vi "Dashboard Main.vi"() -> ()   [LabVIEW 2014]
uses:
  <vilib>/event_ctls.llb/eventvkey.ctl
  <vilib>/Rock Robotics/Network Tables/SD Write Number.vi
  <vilib>/Rock Robotics/WPI/Dashboard/WPI_DashboardLogging Global.vi
  <vilib>/Rock Robotics/Network Tables/SD Read Number.vi
  <vilib>/Utility/config.llb/Write Key (String).vi
  <vilib>/Utility/config.llb/Write Key (I32).vi
  <vilib>/Utility/config.llb/NI_LVConfig.lvlib
panel:
  in  "TCP":refnum<k5>
  in  "Rec Mode":enum32{"Stop", "Record", "Playback"}(radio)
  in  "Vision":u16(ring) items=["Camera Off", "USB Camera SW", "USB Camera HW", "IP Camera"]
  out "Camera IP":string
  out "Image Message":string="Timeout in Camera Communications"
  in  "Dashboard Tab":T1(tab)
  in  "Camera Settings":T2={"Frame Rate"=30, "Compression"=30, "Size"=1} {"Frame Rate" scale=1.0..30.0; "Size" items=["640x480", "320x240", "160x120"]}
  out "MotorChart R":cluster{"Numeric":dbl, "Numeric":dbl}(graph)
  out "MotorChart L":T3(graph)
  out "MotorSliders R":cluster{"MotorSlide1":dbl, "MotorSlide2":dbl} {"MotorSlide2" scale=-1.0..1.0 scale format="%#_2e"; "MotorSlide1" scale=-1.0..1.0 scale format="%#_2e"}
  out "MotorSliders L":T4 {"MotorSlide4 2" scale=0.0..14.0 scale format="%#_2e"; "MotorSlide2" scale=-1.0..1.0 scale format="%#_2e"; "MotorSlide1" scale=-1.0..1.0 scale format="%#_2e"}
  out "Gyro":dbl(knob) scale=0.0..360.0
  out "JS1 Z":dbl(slide) scale=-1.0..1.0 scale format="%#_2e"
  out "JS1 Graph":cluster{"X":dbl, "Y":dbl}[](graph)
  out "JS1 Buttons":T5
  out "JS2 Z":dbl(slide) scale=-1.0..1.0 scale format="%#_2e"
  out "JS2 Graph":cluster{"X":dbl, "Y":dbl}[](graph)
  out "JS2 Buttons":T5
  out "Mode":T6(ring)=enum."Auto Disabled"
  in  "DB Camera Config":bool
  out "fps":dbl format="%#.1g"
  out "Mbps":dbl format="%#.1g"
  out "Mbps 2":bool
  in  "DB/String 9":string
  in  "DB/String 8":string
  in  "DB/String 7":string
  in  "DB/String 6":string
  in  "DB/String 5":string
  in  "DB/String 4":string
  in  "DB/String 3":string
  in  "DB/String 2":string
  in  "DB/String 1":string
  in  "DB/String 0":string
  in  "DB/Slider 0":dbl(slide) scale=0.0..5.0
  in  "DB/Slider 1":dbl(slide) scale=0.0..5.0
  in  "DB/Slider 2":dbl(slide) scale=0.0..5.0
  in  "DB/Slider 3":dbl(slide) scale=0.0..5.0
  out "DB/LED 3":bool
  out "DB/LED 2":bool
  out "DB/LED 1":bool
  out "DB/LED 0":bool
  in  "DB/Button 3":bool
  in  "DB/Button 2":bool
  in  "DB/Button 1":bool
  in  "DB/Button 0":bool caption="New Name"
  out "Guide Box":bool
  in  "a/b":bool
  out "Lift up?":bool
  out "Clasper open?":bool
  out "Clasper closed?":bool
  out "Lift down?":bool
  in  "Autonomous":i32(listbox)
  out "Encoder":dbl(slide) scale=-1.0..1.0 scale format="%#_2e"
  out "Cam Pan":dbl(slide) scale=-1.0..1.0 scale format="%#_2e"
  out "Lift":dbl(slide) scale=-1.0..1.0 scale format="%#_2e"
  out "Cam Tilt":dbl(slide) scale=-1.0..1.0 scale format="%#_2e"
  out "Clasper":dbl(slide) scale=-1.0..1.0 scale format="%#_2e"
  in  "Test Slider":dbl(slide) scale=0.0..100.0 scale format="%#_3g"
  in  "On/Off":bool caption="Solenoid"
  in  "Test Name":u16(ring) items=["Select the test to run...", "Example Test", "-------------------------------", "List of tests is built in robot code.", "Replace with your own automated tests."]
  in  "Test Tree":string(tree)
  in  "Motor":cluster{"Value":dbl, "Enable":bool} {"Value" scale=-1.0..1.0 scale format="%#_3g"}
  out "Progress":T7 {"Test Progress" scale=0.0..100.0}
  in  "Rev/Fwd":cluster{"Forward":bool, "Reverse":bool}
  in  "Test Ring":u16(ring) items=["Monochrome", "Color"]
  in  "Listbox":i32(listbox)
  out "Tree":string(tree)
  out "Camera Image":T8(plugin-control)
  out "Boolean":bool
  # "Left"
  # "Front"
  # "Right"
  # "Battery"
  # "Encoder"
  # "Cam Pan"
  # "Lift"
  # "Cam Tilt"
  # "Clasper"
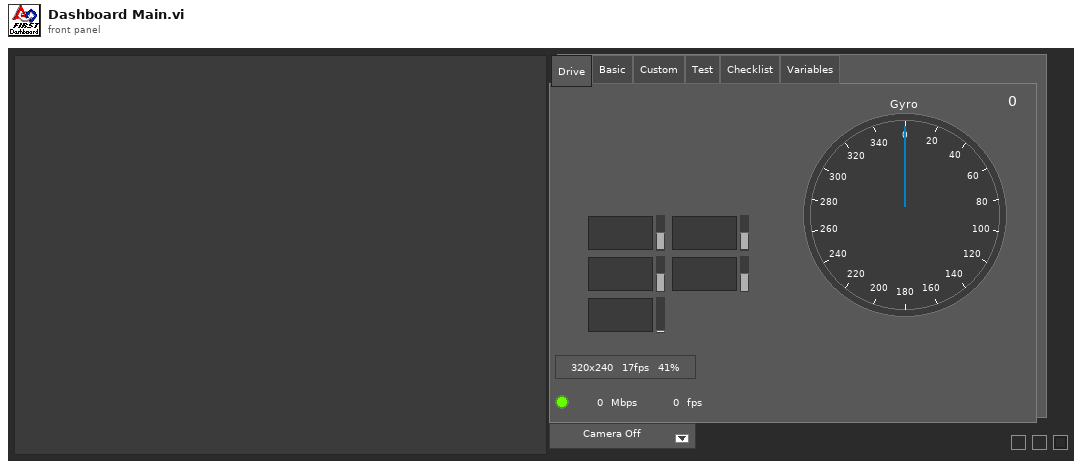
[diagram p1: front panel]
types:
  T1 = enum32{"Drive", "Basic", "Custom", "Test", "Checklist", "Variables"}
  T2 = cluster{"Frame Rate":i32, "Compression":i32, "Size":u16}
  T3 = cluster{"Numeric":dbl, "Numeric":dbl, "Battery V":dbl}
  T4 = cluster{"MotorSlide1":dbl, "MotorSlide2":dbl, "MotorSlide4 2":dbl}
  T5 = cluster{bool, bool, bool, bool, bool, bool, bool, bool, bool, bool, bool, bool}
  T6 = enum8{"Tele-Op Disabled", "Tele-Op Enabled", "Auto Disabled", "Auto Enabled", "Test Disabled", "Test Enabled", "Disconnected", "No Code", "E-Stop"}
  T7 = cluster{"Test Progress":u8, "Test Progress Text":string}
  T8 = typedef "IMAQ Image.ctl" = refnum<image>
  T9 = typedef "Image Type" = u32
  T10 = cluster{"Camera Image":refnum<vi>, "Dashboard Tab":refnum<vi>, "Boolean":refnum<vi>, "Vision":refnum<vi>, "Rec Mode":refnum<vi>, "Test Slider":refnum<vi>, "On/Off ":refnum<vi>, "Test Ring":refnum<vi>, "Rev/Fwd":refnum<vi>, "Test Name":refnum<vi>, "Motor":refnum<vi>, "Progress":refnum<vi>, "CheckList":refnum<vi>, "Tree":refnum<vi>, "Test Tree":refnum<vi>}
  T11 = cluster{"Error Strings":string, "Disable Counts":cluster{u16, u16}, "Rail Faults":cluster{u16, u16, u16}, "Robot IP":string, "DB Mode":u8, "Event Info":cluster{"Name":string, "Type":u8, "Number":u16, "Replay":u8}, "Camera Addr":string}
  T12 = cluster{"Storage":cluster{"Disk Free":u64, "RAM Block":u32, "RAM free":u32}, "CPU Utilization":cluster{"CPU % ISR":sgl, "CPU % Time Crit":sgl, "CPU % Timed Str":sgl, "CPU % High":sgl, "CPU % Above":sgl, "CPU % Normal":sgl, "CPU % Low":sgl}, "CAN":cluster{"% Bus Utilization":sgl, "Bus Off Cnt":u32, "TX_FIFO Full Cnt":u32, "Receive Error Cnt":u8, "Transmit Error Cnt":u8}, "HID":cluster{"HID Outputs":u32, "Rumble Low":u16, "Rumble High":u16}[]}
  T13 = cluster{"Status bits":cluster{"Test Mode":bool, "Autonomous":bool, "Enabled":bool, "Code Start":bool, "Brownout":bool, "Reserved 2":bool, "Reserved 3":bool, "E-Stop":bool}, "Code Trace":cluster{"Disabled":bool, "TeleOp":bool, "Auto":bool, "Test":bool}, "Controller Type":enum16{"unknown", "cRIO", "roboRio"}, "Code?":enum16{"unknown", "noCode", "code"}, "Battery V":dbl}
  T14 = cluster{"Control Bits":cluster{"TestMode":bool, "Autonomous":bool, "Enabled":bool, "FMS Present":bool, bool, bool, bool, "E-Stop":bool}, "Team Station ":u8, "Countdown":sgl, "Joystick Values":cluster{"Axes":dbl[], "Buttons":bool[], "POVs":i16[]}[]}
  T15 = cluster{"Axes":dbl[], "Buttons":bool[], "POVs":i16[]}[]
  T16 = cluster{"Axes":dbl[], "Buttons":bool[], "POVs":i16[]}
  T17 = cluster{"Buttons[0]":bool, "Buttons[1]":bool, "Buttons[2]":bool, "Buttons[3]":bool, "Buttons[4]":bool, "Buttons[5]":bool, "Buttons[6]":bool, "Buttons[7]":bool, "Buttons[8]":bool, "Buttons[9]":bool, "Buttons[10]":bool, "Buttons[11]":bool}
  T18 = typedef "NI_LVConfig.lvlib/Config Data RefNum.ctl" = refnum<k1>
  T19 = cluster{"Operation":enum16{"Update", "Clear"}, "Color Box":u32}[]
  T20 = typedef "eventvkey.ctl" = enum16{"ASCII", "Enter", "Return", "Shift", "Ctrl", "Alt", "Cmd", "Opt", "Caps", "NumLock", "Clear", "Break", "Up", "Down", "Left", "Right", "Insert", "Delete", "Home", "End", "PageUp", "PageDown", "Escape", "Help", "Pause", "ScrollLock", "F1", "F2", "F3", "F4", "F5", "F6", "F7", "F8", "F9", "F10", "F11", "F12", "F13", "F14", "F15", "F16", "F17", "F18", "F19", "F20", "F21", "F22", "F23", "F24", "Play", "VolumeUp", "VolumeDown", "Mute", "Two Byte Char"}
  T21 = cluster{"Image Size":bool, "Image Type":bool, "Pixel Value":bool, "ROI Information":bool, "Zoom Factor":bool}
  T22 = enum8{"Enabled", "Disabled", "Disabled and Grayed Out"}
  T23 = cluster{"Operation":enum16{"Update", "Clear"}, "Color Box":u32}
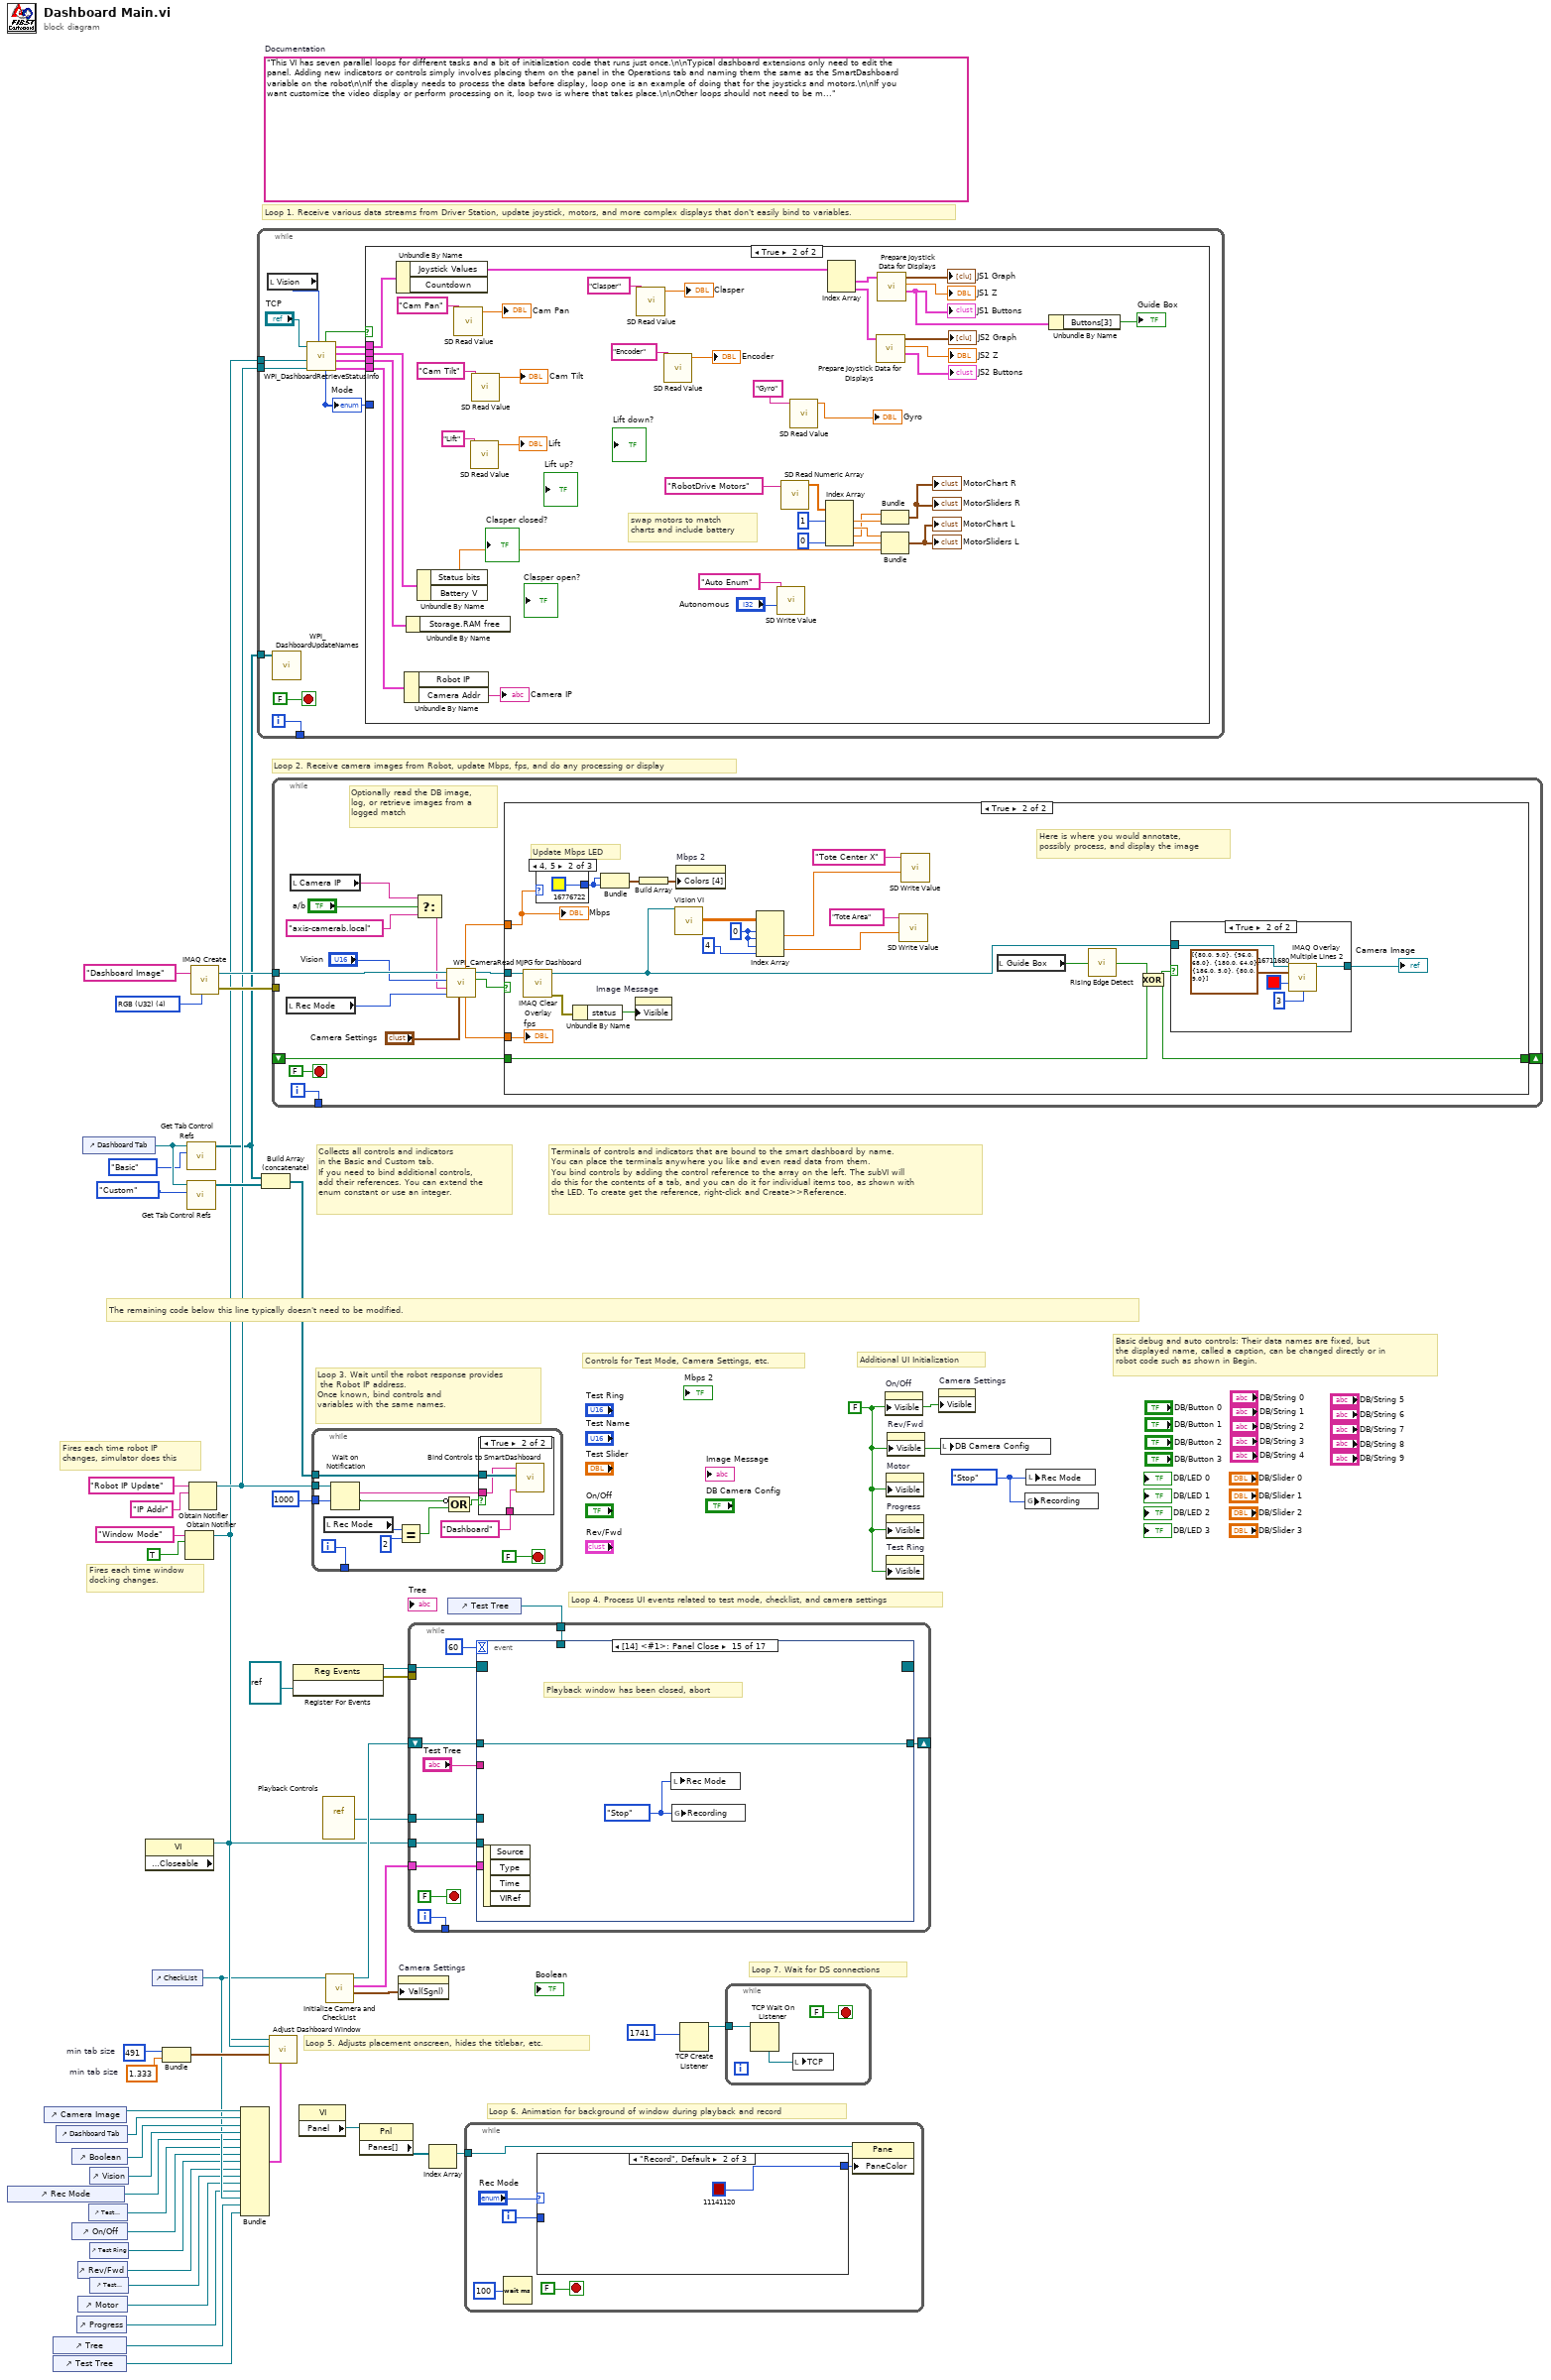
[diagram p0: block diagram]
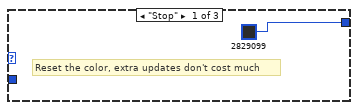
[diagram p3: hidden frame]
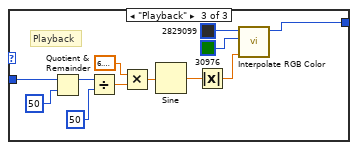
[diagram p4: hidden frame]
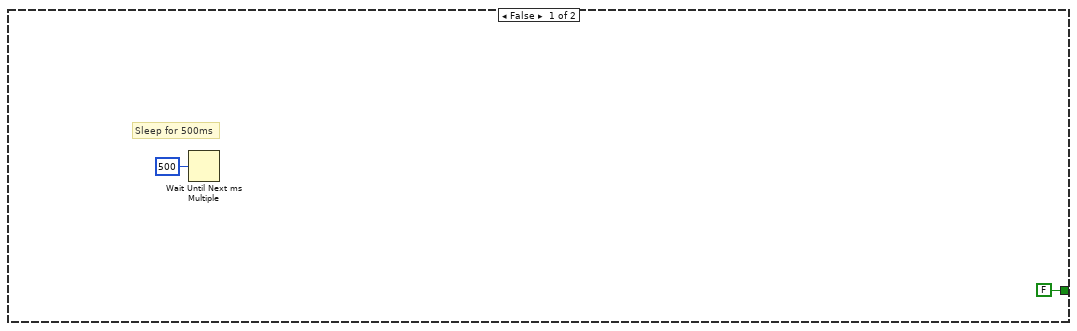
[diagram p6: hidden frame]
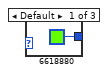
[diagram p8: hidden frame]
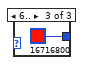
[diagram p9: hidden frame]
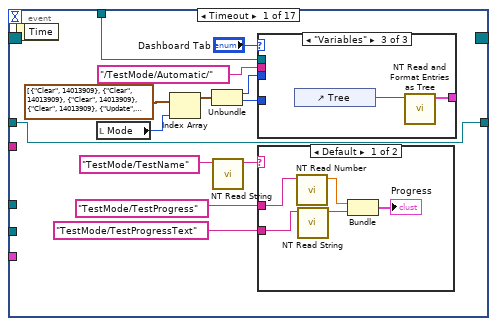
[diagram p10: hidden frame]
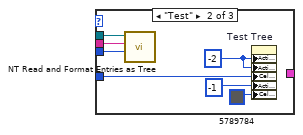
[diagram p12: hidden frame]
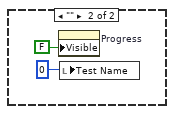
[diagram p13: hidden frame]
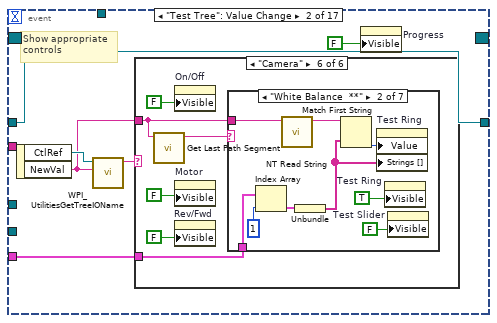
[diagram p14: hidden frame]
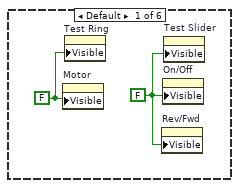
[diagram p15: hidden frame]
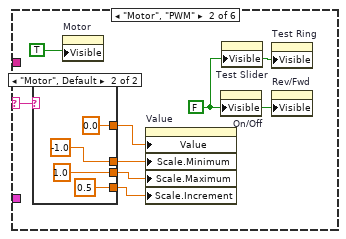
[diagram p16: hidden frame]
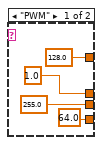
[diagram p17: hidden frame]
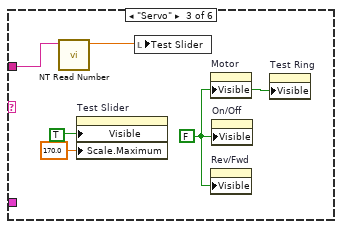
[diagram p18: hidden frame]
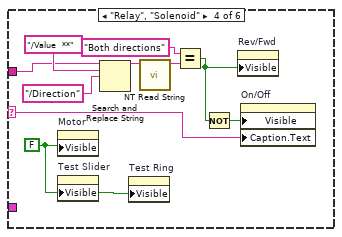
[diagram p19: hidden frame]
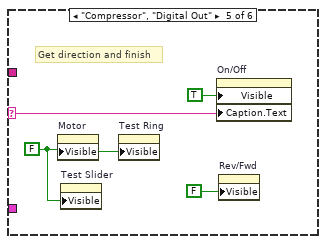
[diagram p20: hidden frame]
diagram:
  w24 = 491  # min tab size
  w23 = 1.333  # min tab size
  w32 = enum32{"Stop", "Record", "Playback"}."Stop" ("Rec Mode")
  w6 = FALSE ("Visible")
  (unwired) "This VI has seven parallel loops for different tasks and a bit of initialization code that runs just once.\n\nTypical dashboard extensions only need to edit the panel. Adding new indicators or controls simply involves placing them on the panel in the Operations tab and naming them the same as the SmartDashboard variable on the robot\n\nIf the display needs to process the data before display, loop one is an example of doing that for the joysticks and motors.\n\nIf you want customize the video display or perform processing on it, loop two is where that takes place.\n\nOther loops should not need to be modified. They are pretty standard, and document the task they perform."  # Documentation
  w52 = T9 4 items=["Grayscale (U8)", "Grayscale (I16)", "Grayscale (SGL)", "Complex (CSG)", "RGB (U32)", "HSL (U32)", "RGB (U64)"] ("Image Type")
  # "Loop 7. Wait for DS connections"
  # "Basic debug and auto controls: Their data names are fixed, but\nthe displayed name, called a caption, can be changed directly or in\nrobot code such as shown in Begin."
  # "Controls for Test Mode, Camera Settings, etc."
  # "Additional UI Initialization"
  # "Loop 6. Animation for background of window during playback and record"
  # "Fires each time robot IP\nchanges, simulator does this"
  # "Fires each time window\ndocking changes."
  # "Collects all controls and indicators\nin the Basic and Custom tab.\nIf you need to bind additional controls,\nadd their references. You can extend the\nenum constant or use an integer."
  # "The remaining code below this line typically doesn't need to be modified."
  # "Loop 4. Process UI events related to test mode, checklist, and camera settings"
  # "Terminals of controls and indicators that are bound to the smart dashboard by name.\nYou can place the terminals anywhere you like and even read data from them.\nYou bind controls by adding the control reference to the array on the left. The subVI will\ndo this for the contents of a tab, and you can do it for individual items too, as shown with\nthe LED. To create get the reference, right-click and Create>>Reference."
  # "Loop 3. Wait until the robot response provides\n the Robot IP address.\nOnce known, bind controls and\nvariables with the same names."
  # "Loop 5. Adjusts placement onscreen, hides the titlebar, etc."
  # "Loop 1. Receive various data streams from Driver Station, update joystick, motors, and more complex displays that don't easily bind to variables."
  # "Loop 2. Receive camera images from Robot, update Mbps, fps, and do any processing or display"
  n1 = control-ref of="Rec Mode"() -> (w12:refnum<vi>)
  n2 = control-ref of="Camera Image"() -> (w27:refnum<vi>)
  n3 = control-ref of="Tree"() -> (w16:refnum<vi>)
  n4 = control-ref of="Test Tree"() -> (w15:refnum<vi>)
  n5 = control-ref of="Dashboard Tab"() -> (w26:refnum<vi>)
  n6 = control-ref of="Boolean"() -> (w21:refnum<vi>)
  n7 = control-ref of="On/Off"() -> (w10:refnum<vi>)
  n8 = control-ref of="Progress"() -> (w7:refnum<vi>)
  n9 = control-ref of="Rev/Fwd"() -> (w8:refnum<vi>)
  n10 = control-ref of="Motor"() -> (w13:refnum<vi>)
  n11 = control-ref of="Dashboard Tab"() -> (w30:refnum<vi>)
  n12 = control-ref of="Test Slider"() -> (w11:refnum<vi>)
  n13 = control-ref of="Vision"() -> (w25:refnum<vi>)
  n14 = control-ref of="Test Ring"() -> (w9:refnum<vi>)
  n15 = control-ref of="Test Name"() -> (w14:refnum<vi>)
  n16 = property class="VI" props=["Front Panel.Closeable"]() -> (reference out=w31:refnum<vi>)  [unwired: 2 in, 2 out]
  n17 = control-ref of="CheckList"() -> (w17:refnum<vi>)
  n18 = Bundle("min tab size"=w24, "min tab size"=w23) -> (w22:cluster{"min tab size":i32, "min tab size":dbl})  [unwired: 1 in]
  n19 = Obtain Notifier(name (unnamed)="Window Mode", notification data type=TRUE) -> (notifier out=w3:refnum<notifier>)  [unwired: 2 in, 2 out]
  n20 = call <vilib>:"Get Tab Control Refs.vi"("Page Index"=T1."Basic" ("Dashboard Tab"), "TabControl in"=w30) -> ("ControlsOnPage"=w4:refnum<vi>[])  [unwired: 9 in]
  n21 = call <vilib>:"Get Tab Control Refs.vi"("Page Index"=T1."Custom" ("Dashboard Tab"), "TabControl in"=w30) -> ("ControlsOnPage"=w29:refnum<vi>[])  [unwired: 9 in]
  n22 = Obtain Notifier(name (unnamed)="Robot IP Update", notification data type="IP Addr" ("name (unnamed)")) -> (notifier out=w5:refnum<notifier>)  [unwired: 2 in, 2 out]
  n23 = call "IMAQ Create"("Image Name"="Dashboard Image", "Image Type"=w52) -> ("New Image"=w50:T8, "error out"=w49:errorcluster)  [unwired: 2 in, 1 out]
  n24 = Bundle("Camera Image"=w27, "Dashboard Tab"=w26, "Boolean"=w21, "Vision"=w25, "Rec Mode"=w12, "Test Slider"=w11, "On/Off"=w10, "Test Ring"=w9, "Rev/Fwd"=w8, "Test Name"=w14, "Motor"=w13, "Progress"=w7, "CheckList"=w17, "Tree"=w16, "Test Tree"=w15) -> (w18:T10)  [unwired: 1 in]
  n25 = while {
    tunnel: [w64] -> _
    tunnel: w5 -> [w58]
    tunnel: w4 -> [w57]
    tunnel: w3 -> [w53]
    i -> [w64]
    stop <- FALSE stop-if-true
    n26 = local read "Vision"() -> (w55:u16)
    n27 = call <vilib>:"WPI_DashboardUpdateNames.vi"("Controls on Tab"=w57) -> ()  [unwired: 11 in]
    n28 = call <vilib>:"WPI_DashboardRetrieveStatusInfo.vi"("Vision"=w55, "Binding Refnum"=w58, "Window Mode Notifier"=w53, "TCP Cnx"="TCP") -> ("Power and Errors"=w59:T11, "Robot Metrics"=w62:T12, "Status Info"=w63:T13, "Control Info"=w60:T14, "Robot Mode"=w56:T6, "Process?"=w61:bool)  [unwired: 2 in]
    "Mode" <- w56
    n29 = case shown="True" w61 {
      tunnel: w63 -> [_ w105]
      tunnel: w62 -> [_ w104]
      tunnel: w60 -> [_ w103]
      tunnel: w59 -> [_ w102]
      tunnel: w56 -> [_ _]
      frame False {
      }
      frame True {
        # "swap motors to match\ncharts and include battery"
        n30 = Unbundle By Name(w103) -> ("Joystick Values"=w81:T15)  [unwired: 1 out]
        n31 = Unbundle By Name(w102) -> ("Camera Addr"=→"Camera IP":string)  [unwired: 1 out]
        n32 = Unbundle By Name(w104) -> ()  [unwired: 1 out]
        n33 = Unbundle By Name(w105) -> ("Battery V"=w92:dbl)  [unwired: 1 out]
        n34 = call-poly <vilib>:"SD Read Value.vi"("Name"="Cam Pan") -> ("Numeric"=→"Cam Pan":dbl)  [unwired: 8 in, 2 out]
        n35 = call-poly <vilib>:"SD Read Value.vi"("Name"="Lift") -> ("Numeric"=→"Lift":dbl)  [unwired: 8 in, 2 out]
        n36 = call-poly <vilib>:"SD Read Value.vi"("Name"="Cam Tilt") -> ("Numeric"=→"Cam Tilt":dbl)  [unwired: 8 in, 2 out]
        n37 = call-poly <vilib>:"SD Read Value.vi"("Name"="Clasper") -> ("Numeric"=→"Clasper":dbl)  [unwired: 8 in, 2 out]
        n38 = call-poly <vilib>:"SD Read Value.vi"("Name"="Encoder") -> ("Numeric"=→"Encoder":dbl)  [unwired: 8 in, 2 out]
        n39 = call-poly <vilib>:"SD Write Value.vi"("Numeric"="Autonomous", "Name"="Auto Enum") -> ()  [unwired: 8 in, 2 out]
        n40 = call <vilib>:"SD Read Numeric Array.vi"("Name"="RobotDrive Motors") -> ("Numeric Array"=w80:dbl[])  [unwired: 8 in, 2 out]
        n41 = call-poly <vilib>:"SD Read Value.vi"("Name"="Gyro") -> ("Numeric"=→"Gyro":dbl)  [unwired: 8 in, 2 out]
        n42 = Index Array(array=w80, index #1=1, index #4=0) -> (element #1=w97:dbl, element #2=w98:dbl, element #3=w96:dbl, element #4=w101:dbl)  [unwired: 2 in]
        n43 = Index Array(array=w81) -> (element #1=w91:T16, element #2=w87:T16)  [unwired: 2 in]
        n44 = call "Prepare Joystick Data for Displays.vi"("Joystick Values"=w87) -> ("Buttons"=→"JS2 Buttons":T17, "Z Axis"=→"JS2 Z":dbl, "Cartesian Data"=→"JS2 Graph":cluster{"X axis":dbl, "X axis":dbl}[])  [unwired: 8 in]
        n45 = call "Prepare Joystick Data for Displays.vi"("Joystick Values"=w91) -> ("Buttons"=w66:T17, "Z Axis"=→"JS1 Z":dbl, "Cartesian Data"=→"JS1 Graph":cluster{"X axis":dbl, "X axis":dbl}[])  [unwired: 8 in]
        "JS1 Buttons" <- w66
        n46 = Bundle("Numeric"=w96, "Numeric"=w97) -> (→"MotorChart R" →"MotorSliders R":cluster{"Numeric":dbl, "Numeric":dbl})  [unwired: 1 in]
        n47 = Bundle("Numeric"=w98, "Numeric"=w101, "Battery V"=w92) -> (→"MotorChart L" →"MotorSliders L":T3)  [unwired: 1 in]
        n48 = Unbundle By Name(w66) -> ("Buttons[3]"=→"Guide Box":bool)
      }
    }
  }
  n49 = Build Array (concatenate)(w4, w29) -> (w28:refnum<vi>[])
  n50 = call "Adjust Dashboard Window.vi"("Sizing Refnums"=w18, "Size Constraints"=w22, "VI"=w31, "Notifier in"=w3) -> ()  [unwired: 8 in]
  n51 = while {
    tunnel: w50 -> [w119]
    tunnel: w49 -> [_]
    tunnel: [w120] -> _
    shift-right: [w107] -> _
    shift-left: _ -> [w106]
    i -> [w120]
    stop <- FALSE stop-if-true
    # "Optionally read the DB image,\nlog, or retrieve images from a\nlogged match"
    n52 = local read "Rec Mode"() -> (w113:enum32{"Stop", "Record", "Playback"})
    n53 = local read "Camera IP"() -> (w109:string)
    n54 = Select(t=w109, s="a/b", f="axis-camerab.local") -> (s? t:f=w108:string)
    n55 = call <vilib>:"WPI_CameraRead MJPG for Dashboard.vi"("Camera Settings"="Camera Settings", "Rec Mode"=w113, "Camera IP"=w108, "Camera Mode"="Vision", "Refnum in"=w119) -> ("Active"=w117:bool, "Refnum out"=w118:T8, "FPS"=w116:dbl, "Bandwidth (Mbps)"=w115:dbl)  [unwired: 3 in]
    n56 = case shown="True" w117 {
      tunnel: w118 -> [_ w139]
      tunnel: w115 -> [_ w138]
      tunnel: w116 -> [_ w137]
      tunnel: [FALSE w129] -> w107
      tunnel: w106 -> [_ w125]
      frame False {
        # "Sleep for 500ms"
        n57 = Wait Until Next ms Multiple(millisecond multiple=u32 500) -> ()  [unwired: 1 out]
      }
      frame True {
        w131 = 0 ("disabled index (row)")
        # "Here is where you would annotate,\npossibly process, and display the image"
        # "Update Mbps LED"
        n58 = call "IMAQ Clear Overlay"("Image"=w139) -> ("error out"=w143:errorcluster, "Image Out"=w124:T8)  [unwired: 2 in, 7 out]
        n59 = case shown="4, 5" w138 {
          tunnel: [u32 6618880 ("Color Box") u32 16776722 ("Color Box") u32 16716800 ("Color Box")] -> w140
          frame Default {
          }
          frame 4, 5 {
          }
          frame 6.. {
          }
        }
        n60 = Unbundle By Name(w143) -> ("status"=w144:bool)
        n61 = Bundle("Color Box"=w140, "Color Box"=w140) -> (w142:cluster{"Color Box":u32, "Color Box":u32})  [unwired: 1 out]
        n62 = property on="Image Message" class="Str"("Visible"=w144) -> ()  [unwired: 2 in, 2 out]
        n63 = Build Array(w142) -> (w141:cluster{"Color Box":u32, "Color Box":u32}[])
        n64 = call "Vision VI.vi"("Image In"=w124) -> ("Particle Measurements (Pixels)"=w136:dbl[][])  [unwired: 24 in, 2 out]
        n65 = property on="Mbps 2" class="Bool (strict)"("Colors [4]"=w141) -> ()  [unwired: 2 in, 2 out]
        n66 = Index Array(array=w136, index (row) #1=w131, index (col) #1=w131, index (row) #2=w131, index (col) #2=4 ("index (row)")) -> (element #1=w130:dbl, element #2=w133:dbl)
        n67 = call-poly <vilib>:"SD Write Value.vi"("Numeric"=w133, "Name"="Tote Area") -> ()  [unwired: 8 in, 2 out]
        n68 = call-poly <vilib>:"SD Write Value.vi"("Numeric"=w130, "Name"="Tote Center X") -> ()  [unwired: 8 in, 2 out]
        n69 = local read "Guide Box"() -> (w127:bool)
        n70 = call "Rising Edge Detect.vi"("Input"=w127) -> ("Output"=w126:bool)
        n71 = Exclusive Or(1:w125, 2:w126) -> (0:w129:bool)
        n72 = case shown="True" w129 {
          tunnel: [w145 w147] -> w128
          tunnel: w124 -> [w145 w146]
          frame False {
          }
          frame True {
            n73 = call "IMAQ Overlay Multiple Lines 2"("Image"=w146, "Line End Points"=cluster{"X":dbl, "Y":dbl}[] [{"X"=80.0, "Y"=9.0}, {"X"=96.0, "Y"=68.0}, {"X"=180.0, "Y"=64.0}, {"X"=186.0, "Y"=5.0}, {"X"=80.0, "Y"=9.0}], "Color"=u32 16711680, "Width"=u32 3) -> ("Image Out"=w147:T8)  [unwired: 10 in, 1 out]
          }
        }
        "Camera Image" <- w128
        "Mbps" <- w138
        "fps" <- w137
      }
    }
  }
  n74 = register-events(refnum<vi> refnum) -> (reference out=w36:refnum<event-registration>, error out=w35:errorcluster)  [unwired: 2 in]
  n75 = property class="VI"() -> ("Panel"=w39:refnum<vi>)  [unwired: 2 in, 2 out]
  n76 = while {
    tunnel: w28 -> [w165]
    tunnel: w5 -> [w163]
    tunnel: [w161] -> _
    tunnel: u32 1000 ("milliseconds to wait") -> [w160]
    i -> [w161]
    stop <- FALSE stop-if-true
    n77 = local read "Rec Mode"() -> (w156:enum32{"Stop", "Record", "Playback"})
    n78 = Wait on Notification(notifier=w163, timeout in ms (-1)=w160) -> (notification=w162:string, timed out?=w158:bool)  [unwired: 2 in, 2 out]
    n79 = Equal?(x=w156, y=u16 2 ("Rec Mode")) -> (x = y?=w157:bool)
    n80 = Compound Arithmetic op=OR(invert w158, w157) -> (w159:bool)
    n81 = case shown="True" w159 {
      tunnel: w165 -> [_ w168]
      tunnel: w162 -> [_ w167]
      tunnel: "Dashboard" -> [_ w166]
      frame False {
      }
      frame True {
        n82 = call <vilib>:"Bind Controls to SmartDashboard.vi"("Client Name"=w166, "Bound Control Refs"=w168, "Server IP Address"=w167) -> ()  [unwired: 9 in]
      }
    }
  }
  n83 = vi-ref "Playback Controls.vi"() -> (w37:refnum<vi>)
  n84 = call "Initialize Camera and CheckList.vi"("ListBox in"=w17) -> ("Cluster"=w43:cluster{"value":i32, "value":i32, "index":i32}, "Array"=w44:cluster{string[]}[], "File Refnum"=w42:T18)  [unwired: 8 in]
  n85 = property class="Pnl"(reference=w39) -> ("Panes[]"=w40:refnum<vi>[])  [unwired: 1 in, 2 out]
  n86 = property on="Camera Settings" class="Clust (strict)"("Val(Sgnl)"=w43) -> ()  [unwired: 2 in, 2 out]
  n87 = Index Array(array=w40) -> (element=w38:refnum<vi>)  [unwired: 1 in]
  n88 = control-ref of="Test Tree"() -> (w41:refnum<vi>)
  n89 = while {
    tunnel: w44 -> [w176]
    shift-right: [w175] -> _
    shift-left: w42 -> [w174]
    tunnel: [w173] -> _
    tunnel: w41 -> [w172]
    tunnel: w37 -> [w171]
    tunnel: w36 -> [w170]
    tunnel: w35 -> [_]
    tunnel: w31 -> [w169]
    i -> [w173]
    stop <- FALSE stop-if-true
    n90 = event shown="[14] <#1>: Panel Close" {
      selector: w170 -> [_ _ _ _ _ _ _ _ _ _ _ _ _ _ _ _ _]
      dyn-events: [_ _ _ _ _ _ _ _ _ _ _ _ _ w414 _ _ _] -> _
      timeout: u32 60 ("milliseconds to wait") -> [_ _ _ _ _ _ _ _ _ _ _ _ _ _ _ _ _]
      tunnel: w172 -> [w188 _ _ _ _ _ _ _ _ _ _ _ _ _ _ _ _]
      tunnel: "Test Tree" -> [_ _ _ _ _ _ _ _ w383 w391 w393 w397 w405 _ _ _ _]
      tunnel: w176 -> [_ w210 _ _ _ _ w347 w377 _ _ _ _ _ _ _ _ _]
      tunnel: [w184 w209 w308 w313 w321 w333 w346 w370 w382 w389 w392 w396 w404 w416 w430 w431 w441] -> w175
      tunnel: w174 -> [w184 w209 w308 w313 w321 w333 w345 w370 w382 w389 w392 w396 w404 w416 w430 w431 w441]
      tunnel: w171 -> [_ _ _ _ _ _ _ _ _ _ _ _ _ w417 _ w434 _]
      tunnel: w169 -> [_ _ _ _ _ _ _ _ _ _ _ _ _ w412 _ _ _]
      event Timeout {
        n91 = event-data() -> ()  [unwired: 1 in, 1 out]
        n92 = local read "Mode"() -> (w187:T6)
        n93 = Index Array(array=T19 [{"Operation"=enum."Clear", "Color Box"=14013909}, {"Operation"=enum."Clear", "Color Box"=14013909}, {"Operation"=enum."Clear", "Color Box"=14013909}, {"Operation"=enum."Clear", "Color Box"=14013909}, {"Operation"=enum."Update", "Color Box"=14013909}, {"Operation"=enum."Update", "Color Box"=16777215}, {"Operation"=enum."Clear", "Color Box"=14013909}, {"Operation"=enum."Clear", "Color Box"=14013909}, {"Operation"=enum."Clear", "Color Box"=14013909}], index=w187) -> (element=w182:T23)
        n94 = Unbundle(w182) -> ("Operation"=w181:enum16{"Update", "Clear"}, "Color Box"=w180:u32)
        n95 = call <vilib>:"NT Read String.vi"("Name"="TestMode/TestName") -> ("String"=w191:string)  [unwired: 9 in, 1 out]
        n96 = case shown="\"Variables\"" "Dashboard Tab" {
          tunnel: w188 -> [_ w199 _]
          tunnel: "/TestMode/Automatic/" ("Name Pattern") -> [_ w198 _]
          tunnel: w181 -> [_ w197 _]
          tunnel: [_ _ w201] -> _
          tunnel: w180 -> [_ w193 _]
          frame "Custom", Default {
          }
          frame "Test" {
            w196 = -2 ("Active Item:Row Number")
            n97 = call <vilib>:"NT Read and Format Entries as Tree.vi"("Operation"=w197, "Name Pattern"=w198, "Tree Refnum"=w199) -> ()  [unwired: 7 in, 2 out]
            n98 = property on="Test Tree" class="Tree (strict)"("Active Item Row Number"=w196, "ActiveColNum"=w196, "CellBG"=w193, "Active Item Row Number"=-1 ("Active Item:Row Number"), "CellBG"=u32 5789784 ("Color Box")) -> ()  [unwired: 2 in, 2 out]
          }
          frame "Variables" {
            n99 = control-ref of="Tree"() -> (w200:refnum<vi>)
            n100 = call <vilib>:"NT Read and Format Entries as Tree.vi"("Tree Refnum"=w200) -> ("Formatted Strings"=w201:cluster{"Name":string, "Value":string}[])  [unwired: 9 in, 1 out]
          }
        }
        n101 = case shown="Default" w191 {
          tunnel: "TestMode/TestProgress" ("Name") -> [w203 _]
          tunnel: "TestMode/TestProgressText" ("Name") -> [w202 _]
          frame Default {
            n102 = call <vilib>:"NT Read Number.vi"("Name"=w203) -> ("Numeric"=w204:dbl)  [unwired: 9 in, 1 out]
            n103 = call <vilib>:"NT Read String.vi"("Name"=w202) -> ("String"=w205:string)  [unwired: 9 in, 1 out]
            n104 = Bundle("Numeric"=w204, "String"=w205) -> (→"Progress":cluster{"Numeric":dbl, "String":string})  [unwired: 1 in]
          }
          frame "" {
            n105 = property on="Progress" class="Clust (strict)"("Visible"=FALSE) -> ()  [unwired: 2 in, 2 out]
            n106 = local write "Test Name"(u16 0) -> ()
          }
        }
      }
      event "Test Tree": Value Change {
        # "Show appropriate\ncontrols"
        n107 = event-data() -> ("CtlRef"=w213:refnum<vi>, "NewVal"=w211:string)  [unwired: 1 in]
        n108 = call <vilib>:"WPI_UtilitiesGetTreeIOName.vi"("NewVal"=w211, "TreeControl in"=w213) -> ("I/O Name"=w214:string)  [unwired: 9 in]
        n109 = case shown="\"Camera\"" w214 {
          selector: w214 -> [_ w221 _ w239 w248 _]
          tunnel: w211 -> [_ _ w236 w238 _ w255]
          tunnel: w210 -> [_ _ _ _ _ w254]
          frame Default {
            w216 = FALSE ("Visible")
            w215 = FALSE ("Visible")
            n110 = property on="Motor" class="Clust (strict)"("Visible"=w215) -> ()  [unwired: 2 in, 2 out]
            n111 = property on="Test Ring" class="Ring (strict)"("Visible"=w215) -> ()  [unwired: 2 in, 2 out]
            n112 = property on="Rev/Fwd" class="Clust (strict)"("Visible"=w216) -> ()  [unwired: 2 in, 2 out]
            n113 = property on="On/Off" class="Bool (strict)"("Visible"=w216) -> ()  [unwired: 2 in, 2 out]
            n114 = property on="Test Slider" class="Slide (strict)"("Visible"=w216) -> ()  [unwired: 2 in, 2 out]
          }
          frame "Motor", "PWM" {
            w222 = FALSE ("Visible")
            n115 = case shown="\"Motor\", Default" w221 {
              tunnel: [1.0 ("Value") -1.0 ("Value")] -> w220
              tunnel: [255.0 ("Value") 1.0 ("Value")] -> w219
              tunnel: [128.0 ("Value") 0.0 ("Value")] -> w218
              tunnel: [64.0 ("Value") 0.5 ("Value")] -> w217
              frame "PWM" {
              }
              frame "Motor", Default {
              }
            }
            n116 = property on="Motor" class="Clust (strict)"("Visible"=TRUE) -> ()  [unwired: 2 in, 2 out]
            n117 = property on="Value" class="Slide (strict)"("Value"=w218, "Scale.Minimum"=w220, "Scale.Maximum"=w219, "Scale.Increment"=w217) -> ()  [unwired: 2 in, 2 out]
            n118 = property on="On/Off" class="Bool (strict)"("Visible"=w222) -> ()  [unwired: 2 in, 2 out]
            n119 = property on="Test Slider" class="Slide (strict)"("Visible"=w222) -> ()  [unwired: 2 in, 2 out]
            n120 = property on="Test Ring" class="Ring (strict)"("Visible"=w222) -> ()  [unwired: 2 in, 2 out]
            n121 = property on="Rev/Fwd" class="Clust (strict)"("Visible"=w222) -> ()  [unwired: 2 in, 2 out]
          }
          frame "Servo" {
            w234 = FALSE ("Visible")
            n122 = call <vilib>:"NT Read Number.vi"("Name"=w236) -> ("Numeric"=w235:dbl)  [unwired: 9 in, 1 out]
            n123 = property on="Test Slider" class="Slide (strict)"("Visible"=TRUE, "Scale.Maximum"=170.0 ("Scale.Range:Maximum")) -> ()  [unwired: 2 in, 2 out]
            n124 = local write "Test Slider"(w235) -> ()
            n125 = property on="Motor" class="Clust (strict)"("Visible"=w234) -> ()  [unwired: 2 in, 2 out]
            n126 = property on="Rev/Fwd" class="Clust (strict)"("Visible"=w234) -> ()  [unwired: 2 in, 2 out]
            n127 = property on="On/Off" class="Bool (strict)"("Visible"=w234) -> ()  [unwired: 2 in, 2 out]
            n128 = property on="Test Ring" class="Ring (strict)"("Visible"=w234) -> ()  [unwired: 2 in, 2 out]
          }
          frame "Relay", "Solenoid" {
            w237 = FALSE ("Visible")
            n129 = property on="Motor" class="Clust (strict)"("Visible"=w237) -> ()  [unwired: 2 in, 2 out]
            n130 = property on="Test Slider" class="Slide (strict)"("Visible"=w237) -> ()  [unwired: 2 in, 2 out]
            n131 = Search and Replace String(input string=w238, search string="/Value  **", replace string="/Direction") -> (result string=w244:string)  [unwired: 5 in, 3 out]
            n132 = property on="Test Ring" class="Ring (strict)"("Visible"=w237) -> ()  [unwired: 2 in, 2 out]
            n133 = call <vilib>:"NT Read String.vi"("Name"=w244) -> ("String"=w242:string)  [unwired: 9 in, 1 out]
            n134 = Equal?(x="Both directions", y=w242) -> (x = y?=w240:bool)
            n135 = Not(x=w240) -> (.not. x?=w241:bool)
            n136 = property on="Rev/Fwd" class="Clust (strict)"("Visible"=w240) -> ()  [unwired: 2 in, 2 out]
            n137 = property on="On/Off" class="Bool (strict)"("Visible"=w241, "Caption.Text"=w239) -> ()  [unwired: 2 in, 2 out]
          }
          frame "Compressor", "Digital Out" {
            w247 = FALSE ("Visible")
            # "Get direction and finish"
            n138 = property on="Motor" class="Clust (strict)"("Visible"=w247) -> ()  [unwired: 2 in, 2 out]
            n139 = property on="Test Slider" class="Slide (strict)"("Visible"=w247) -> ()  [unwired: 2 in, 2 out]
            n140 = property on="Test Ring" class="Ring (strict)"("Visible"=w247) -> ()  [unwired: 2 in, 2 out]
            n141 = property on="On/Off" class="Bool (strict)"("Visible"=TRUE, "Caption.Text"=w248) -> ()  [unwired: 2 in, 2 out]
            n142 = property on="Rev/Fwd" class="Clust (strict)"("Visible"=FALSE) -> ()  [unwired: 2 in, 2 out]
          }
          frame "Camera" {
            n143 = call <vilib>:"Get Last Path Segment.vi"("String in"=w255) -> ("String out"=w256:string)  [unwired: 10 in]
            n144 = property on="On/Off" class="Bool (strict)"("Visible"=FALSE) -> ()  [unwired: 2 in, 2 out]
            n145 = property on="Motor" class="Clust (strict)"("Visible"=FALSE) -> ()  [unwired: 2 in, 2 out]
            n146 = property on="Rev/Fwd" class="Clust (strict)"("Visible"=FALSE) -> ()  [unwired: 2 in, 2 out]
            n147 = case shown="\"White Balance  **\"" w256 {
              tunnel: w255 -> [w262 w271 w280 w289 w298 _ w304]
              tunnel: w254 -> [w260 w268 w277 w286 w295 _ _]
              frame "Size  **" {
                n148 = Index Array(array=w260) -> (element=w259:cluster{string[]})  [unwired: 1 in]
                n149 = call <vilib>:"NT Read String.vi"("Name"=w262) -> ("String"=w261:string)  [unwired: 9 in, 1 out]
                n150 = Unbundle(w259) -> (w257:string[])
                n151 = Match First String(2:w257, 3:w261) -> (0:w258:i32)  [unwired: 1 out]
                n152 = property on="Test Ring" class="Ring (strict)"("Value"=w258, "Strings []"=w257) -> ()  [unwired: 2 in, 2 out]
                n153 = property on="Test Ring" class="Ring (strict)"("Visible"=TRUE) -> ()  [unwired: 2 in, 2 out]
                n154 = property on="Test Slider" class="Slide (strict)"("Visible"=FALSE) -> ()  [unwired: 2 in, 2 out]
              }
              frame "White Balance  **" {
                n155 = Index Array(array=w268, index=1) -> (element=w269:cluster{string[]})
                n156 = call <vilib>:"NT Read String.vi"("Name"=w271) -> ("String"=w270:string)  [unwired: 9 in, 1 out]
                n157 = Unbundle(w269) -> (w266:string[])
                n158 = Match First String(2:w266, 3:w270) -> (0:w265:i32)  [unwired: 1 out]
                n159 = property on="Test Ring" class="Ring (strict)"("Value"=w265, "Strings []"=w266) -> ()  [unwired: 2 in, 2 out]
                n160 = property on="Test Ring" class="Ring (strict)"("Visible"=TRUE) -> ()  [unwired: 2 in, 2 out]
                n161 = property on="Test Slider" class="Slide (strict)"("Visible"=FALSE) -> ()  [unwired: 2 in, 2 out]
              }
              frame "Exposure  **" {
                n162 = Index Array(array=w277, index=2) -> (element=w278:cluster{string[]})
                n163 = call <vilib>:"NT Read String.vi"("Name"=w280) -> ("String"=w279:string)  [unwired: 9 in, 1 out]
                n164 = Unbundle(w278) -> (w274:string[])
                n165 = Match First String(2:w274, 3:w279) -> (0:w275:i32)  [unwired: 1 out]
                n166 = property on="Test Ring" class="Ring (strict)"("Value"=w275, "Strings []"=w274) -> ()  [unwired: 2 in, 2 out]
                n167 = property on="Test Ring" class="Ring (strict)"("Visible"=TRUE) -> ()  [unwired: 2 in, 2 out]
                n168 = property on="Test Slider" class="Slide (strict)"("Visible"=FALSE) -> ()  [unwired: 2 in, 2 out]
              }
              frame "Exposure Priority  **" {
                n169 = Index Array(array=w286, index=3) -> (element=w287:cluster{string[]})
                n170 = call <vilib>:"NT Read String.vi"("Name"=w289) -> ("String"=w288:string)  [unwired: 9 in, 1 out]
                n171 = Unbundle(w287) -> (w283:string[])
                n172 = Match First String(2:w283, 3:w288) -> (0:w284:i32)  [unwired: 1 out]
                n173 = property on="Test Ring" class="Ring (strict)"("Value"=w284, "Strings []"=w283) -> ()  [unwired: 2 in, 2 out]
                n174 = property on="Test Ring" class="Ring (strict)"("Visible"=TRUE) -> ()  [unwired: 2 in, 2 out]
                n175 = property on="Test Slider" class="Slide (strict)"("Visible"=FALSE) -> ()  [unwired: 2 in, 2 out]
              }
              frame "Color Enable  **" {
                n176 = Index Array(array=w295, index=4) -> (element=w296:cluster{string[]})
                n177 = call <vilib>:"NT Read String.vi"("Name"=w298) -> ("String"=w297:string)  [unwired: 9 in, 1 out]
                n178 = Unbundle(w296) -> (w292:string[])
                n179 = Match First String(2:w292, 3:w297) -> (0:w293:i32)  [unwired: 1 out]
                n180 = property on="Test Ring" class="Ring (strict)"("Value"=w293, "Strings []"=w292) -> ()  [unwired: 2 in, 2 out]
                n181 = property on="Test Ring" class="Ring (strict)"("Visible"=TRUE) -> ()  [unwired: 2 in, 2 out]
                n182 = property on="Test Slider" class="Slide (strict)"("Visible"=FALSE) -> ()  [unwired: 2 in, 2 out]
              }
              frame Default {
                n183 = property on="Test Ring" class="Ring (strict)"("Visible"=FALSE) -> ()  [unwired: 2 in, 2 out]
                n184 = property on="Test Slider" class="Slide (strict)"("Visible"=FALSE) -> ()  [unwired: 2 in, 2 out]
              }
              frame "Brightness  **", "Color Level  **", "Compression  **", "FPS  **", "Sharpness  **" {
                n185 = call <vilib>:"NT Read Number.vi"("Name"=w304) -> ("Numeric"=w303:dbl)  [unwired: 9 in, 1 out]
                n186 = local write "Test Slider"(w303) -> ()
                n187 = property on="Test Slider" class="Slide (strict)"("Visible"=TRUE, "Scale.Maximum"=100.0 ("Scale.Range:Maximum")) -> ()  [unwired: 2 in, 2 out]
                n188 = property on="Test Ring" class="Ring (strict)"("Visible"=FALSE) -> ()  [unwired: 2 in, 2 out]
              }
            }
          }
        }
        n189 = property on="Progress" class="Clust (strict)"("Visible"=FALSE) -> ()  [unwired: 2 in, 2 out]
      }
      event "Test Name": Mouse Enter {
        # "Populate the ring with the list of tests"
        n190 = event-data() -> ()  [unwired: 1 in, 1 out]
        n191 = call <vilib>:"NT Read String Array.vi"("Name"="TestMode/TestList") -> ("String Array"=w312:string[])  [unwired: 9 in, 1 out]
        n192 = Build Array (concatenate)("Select the test to run...", w312) -> (w311:string[])
        n193 = property on="Test Name" class="Ring (strict)"("Strings []"=w311) -> ()  [unwired: 2 in, 2 out]
      }
      event "Test Name": Value Change {
        w314 = FALSE ("Visible")
        # "Tell the robot the test name to run"
        n194 = event-data() -> ("NewVal"=w318:u16)  [unwired: 1 in]
        n195 = property on="Test Name" class="Ring (strict)"() -> ("Strings []"=w319:string[])  [unwired: 2 in, 2 out]
        n196 = local write "Progress"(T7 {"Test Progress"=0, "Test Progress Text"=""} ("Progress")) -> ()
        n197 = Index Array(array=w319, index=w318) -> (element=w317:string)
        n198 = call <vilib>:"NT Write String.vi"("String"=w317, "Name"="TestMode/TestName") -> ()  [unwired: 9 in, 1 out]
        n199 = property on="Progress" class="Clust (strict)"("Visible"=TRUE) -> ()  [unwired: 2 in, 2 out]
        n200 = property on="Motor" class="Clust (strict)"("Visible"=w314) -> ()  [unwired: 2 in, 2 out]
        n201 = property on="Test Slider" class="Slide (strict)"("Visible"=w314) -> ()  [unwired: 2 in, 2 out]
        n202 = property on="On/Off" class="Bool (strict)"("Visible"=w314) -> ()  [unwired: 2 in, 2 out]
        n203 = property on="Rev/Fwd" class="Clust (strict)"("Visible"=w314) -> ()  [unwired: 2 in, 2 out]
        n204 = property on="Test Ring" class="Ring (strict)"("Visible"=w314) -> ()  [unwired: 2 in, 2 out]
      }
      event "Listbox": Double Click {
        # "Shift clears all"
        # "Update symbols on the listbox"
        n205 = event-data() -> ("PlatMods.Shift"=w322:bool, "Row"=w324:i32)  [unwired: 1 in]
        n206 = case shown="True" w322 {
          tunnel: w324 -> [w328 _]
          tunnel: 1 -> [w327 _]
          frame False {
            n207 = property on="Listbox" class="LstBox (strict)"() -> ("Item Symbols"=w326:i32[])  [unwired: 2 in, 2 out]
            n208 = Replace Array Subset(array=w326, new element=w327, index=w328) -> (w325:i32[])
            n209 = property on="Listbox" class="LstBox (strict)"("Item Symbols"=w325) -> ()  [unwired: 2 in, 2 out]
          }
          frame True {
            w329 = 0 ("Top Row")
            n210 = property on="Listbox" class="LstBox (strict)"() -> ("Number of Rows"=w331:u32)  [unwired: 2 in, 2 out]
            n211 = Initialize Array(0, w331) -> (w330:i32[])
            n212 = property on="Listbox" class="LstBox (strict)"("Top Row"=w329, "Value"=w329, "Item Symbols"=w330) -> ()  [unwired: 2 in, 2 out]
          }
        }
      }
      event "Listbox": Key Down {
        # "Update symbols on the listbox\nLeft and right keys check and uncheck"
        n213 = event-data() -> ("VKey"=w335:T20)  [unwired: 1 in]
        n214 = case shown="\"Left\", \"Right\"" w335 {
          selector: w335 -> [w340 _]
          tunnel: eventvkey."Left" ("VKey") -> [w338 _]
          frame "Left", "Right" {
            n215 = Equal?(x=w338, y=w340) -> (x = y?=w339:bool)
            n216 = Select(t=0, s=w339, f=1) -> (s? t:f=w341:i32)
            n217 = property on="Listbox" class="LstBox (strict)"() -> ("Item Symbols"=w344:i32[])  [unwired: 2 in, 2 out]
            n218 = Replace Array Subset(array=w344, new element=w341, index="Listbox") -> (w343:i32[])
            n219 = property on="Listbox" class="LstBox (strict)"("Item Symbols"=w343) -> ()  [unwired: 2 in, 2 out]
          }
          frame Default {
          }
        }
      }
      event "DB Camera Config": Value Change {
        # "Show or hide the cluster of controls, store in ini file"
        n220 = event-data() -> ("NewVal"=w348:bool)  [unwired: 1 in]
        n221 = case shown="False" w348 {
          tunnel: w347 -> [w357 _]
          tunnel: [w350 w368] -> w346
          tunnel: w345 -> [w349 w368]
          frame False {
            w364 = "Camera"
            w367 = FALSE ("Visible")
            n222 = local read "Camera Settings"() -> (w356:T2)
            n223 = Index Array(array=w357) -> (element=w360:cluster{string[]})  [unwired: 1 in]
            n224 = Unbundle(w356) -> ("Frame Rate"=w355:i32, "Compression"=w354:i32, "Size"=w358:u16)
            n225 = Unbundle(w360) -> (w359:string[])
            n226 = Index Array(array=w359, index=w358) -> (element=w353:string)
            n227 = call-poly <vilib>:"Write Key.vi"("section"=w364, "value"=w353, "key"="Size", "refnum"=w349) -> ("refnum out"=w366:T18)  [unwired: 2 in, 5 out]
            n228 = call-poly <vilib>:"Write Key.vi"("section"=w364, "value"=w355, "key"="FrameRate", "refnum"=w366) -> ("refnum out"=w365:T18)  [unwired: 1 in, 6 out]
            n229 = property on="Camera Settings" class="Clust (strict)"("Visible"=w367) -> ()  [unwired: 2 in, 2 out]
            n230 = local write "DB Camera Config"(w367) -> ()
            n231 = call-poly <vilib>:"Write Key.vi"("section"=w364, "value"=w354, "key"="Compression", "refnum"=w365) -> ("refnum out"=w351:T18)  [unwired: 1 in, 6 out]
            n232 = call <vilib>:"Close Config Data.vi"("refnum"=w351) -> ("file path"=w352:path)  [unwired: 2 in, 8 out]
            n233 = call <vilib>:"Open Config Data.vi"("configuration file path"=w352) -> ("refnum"=w350:T18)  [unwired: 8 in, 2 out]
          }
          frame True {
            n234 = property on="Camera Settings" class="Clust (strict)"("Visible"=TRUE) -> ()  [unwired: 2 in, 2 out]
          }
        }
      }
      event "Camera Settings": Value Change {
        # "Update summary string when any elements of DB camera change"
        n235 = event-data() -> ("NewVal"=w381:T2)  [unwired: 1 in]
        n236 = Index Array(array=w377) -> (element=w376:cluster{string[]})  [unwired: 1 in]
        n237 = Unbundle(w381) -> ("Frame Rate"=w372:i32, "Compression"=w371:i32, "Size"=w374:u16)
        n238 = Unbundle(w376) -> (w375:string[])
        n239 = Index Array(array=w375, index=w374) -> (element=w373:string)
        n240 = Format Into String(format string="%s   %dfps   %d%%", w373, w372, w371) -> (resulting string=w378:string)  [unwired: 2 in, 1 out]
        n241 = Build Array(w378) -> (w379:string[])
        n242 = property on="DB Camera Config" class="Bool (strict)"("Strings [4]"=w379) -> ()  [unwired: 2 in, 2 out]
      }
      event "Motor.Enable": Value Change {
        # "When the test mode otor enable helper is set, update that\ntree row item's value"
        n243 = event-data() -> ("NewVal"=w387:bool)  [unwired: 1 in]
        n244 = Unbundle("Motor") -> ("Value"=w386:dbl)  [unwired: 1 out]
        n245 = Select(t=w386, s=w387, f=0.0) -> (s? t:f=w384:dbl)
        n246 = call <vilib>:"NT Write Number.vi"("Numeric"=w384, "Name"=w383) -> ()  [unwired: 9 in, 1 out]
      }
      event "Test Slider": Value Change {
        # "When the test mode slider helper is set, update that\ntree row item's value"
        n247 = event-data() -> ("NewVal"=w390:dbl)  [unwired: 1 in]
        n248 = call <vilib>:"NT Write Number.vi"("Numeric"=w390, "Name"=w391) -> ()  [unwired: 9 in, 1 out]
      }
      event "On/Off": Value Change {
        # "When the test mode on/off helper value is set, update that\ntree row item's value"
        n249 = event-data() -> ("NewVal"=w395:bool)  [unwired: 1 in]
        n250 = Boolean To (0,1)(Boolean=w395) -> (0, 1=w394:i16)
        n251 = call <vilib>:"NT Write Number.vi"("Numeric"=w394, "Name"=w393) -> ()  [unwired: 9 in, 1 out]
      }
      event "Rev/Fwd": Value Change {
        # "When the test mode helper value for relays is set, update that\ntree row item's value"
        n252 = event-data() -> ("NewVal.Forward"=w403:bool, "NewVal.Reverse"=w402:bool)  [unwired: 1 in]
        n253 = Boolean To (0,1)(Boolean=w403) -> (0, 1=w399:i16)
        n254 = Boolean To (0,1)(Boolean=w402) -> (0, 1=w401:i16)
        n255 = Negate(x=w401) -> (-x=w400:i16)
        n256 = Add(x=w399, y=w400) -> (x+y=w398:i16)
        n257 = call <vilib>:"NT Write Number.vi"("Numeric"=w398, "Name"=w397) -> ()  [unwired: 9 in, 1 out]
      }
      event "Test Ring": Value Change {
        # "When a test mode helper value is selected from the ring,\nset the tree item's variable to the string value"
        n258 = event-data() -> ("NewVal"=w407:u16)  [unwired: 1 in]
        n259 = property on="Test Ring" class="Ring (strict)"() -> ("Strings []"=w408:string[])  [unwired: 2 in, 2 out]
        n260 = Index Array(array=w408, index=w407) -> (element=w406:string)
        n261 = call <vilib>:"NT Write String.vi"("String"=w406, "Name"=w405) -> ()  [unwired: 9 in, 1 out]
      }
      event "Rec Mode": Value Change {
        # "Update globals for recording mode and path to read log from.\nClear when logging and let NetworkTables set path for vision to\nuse."
        n262 = event-data() -> ("NewVal"=w418:enum32{"Stop", "Record", "Playback"})  [unwired: 1 in]
        n263 = global write "WPI_DashboardLogging Global.vi" "Logging Filename"(path "") -> ()
        n264 = case shown="\"Playback\"" w418 {
          tunnel: w417 -> [_ w420 w428]
          tunnel: [_ _ w427] -> w414
          tunnel: [_ _ w426] -> _
          tunnel: w412 -> [_ _ w424]
          tunnel: cluster{i32, i32} {-250, 170} -> [_ _ w423]
          tunnel: [_ _ T21 {"Image Size"=TRUE, "Image Type"=TRUE, "Pixel Value"=TRUE, "ROI Information"=TRUE, "Zoom Factor"=FALSE} ("Image Information Shown:All Elements")] -> w410
          tunnel: [_ _ TRUE ("Zoom Factor")] -> w409
          frame Default {
          }
          frame "Stop", "Record" {
            # "Place Window too"
            n265 = invoke class="VI" method="FP.Close"(reference=w420) -> (reference out=w419:refnum<vi>)  [unwired: 2 in, 2 out]
            n266 = invoke class="VI" method="Abort VI"(reference=w419) -> ()  [unwired: 2 in, 3 out]
          }
          frame "Playback" {
            n267 = call "Open Playback Panel.vi"("Offset"=w423, "DB VI Ref"=w424, "Playback in"=w428) -> ("Playback out"=w425:refnum<vi>)  [unwired: 8 in]
            n268 = register-events(w425) -> (reference out=w427:refnum<event-registration>, error out=w426:errorcluster)  [unwired: 2 in]
          }
        }
        n269 = global write "WPI_DashboardLogging Global.vi" "Recording"(w418) -> ()
        n270 = property on="Camera Image" class="ImageControl"("Image Information Shown"=w410, "Image Information Visible"=w409) -> ()  [unwired: 2 in, 2 out]
        n271 = call <vilib>:"WPI_DashboardNT Log FieldName Cache.vi"("Operation"=enum16{"Lookup/Add", "Index", "Clear"}."Clear") -> ()  [unwired: 8 in, 3 out]
      }
      event Panel Close {
        w429 = enum32{"Stop", "Record", "Playback"}."Stop" ("Rec Mode")
        # "Playback window has been closed, abort"
        n272 = event-data() -> ()  [unwired: 1 in, 4 out]
        n273 = local write "Rec Mode"(w429) -> ()
        n274 = global write "WPI_DashboardLogging Global.vi" "Recording"(w429) -> ()
      }
      event Panel Close {
        # "Abort playback window and ourself"
        n275 = event-data() -> ()  [unwired: 1 in, 4 out]
        n276 = invoke class="VI" method="FP.Close"(reference=w434) -> (reference out=w433:refnum<vi>)  [unwired: 2 in, 2 out]
        n277 = invoke class="VI" method="Abort VI"(reference=w433) -> (error out=w432:errorcluster)  [unwired: 2 in, 2 out]
        n278 = invoke class="VI" method="Abort VI"(error in=w432) -> ()  [unwired: 2 in, 3 out]
      }
      event "Vision": Value Change {
        # "Enable/Disable Compression slider.\nHW USB is hard-coded into the camera"
        n279 = event-data() -> ("NewVal"=w440:u16)  [unwired: 1 in]
        n280 = Equal?(x=w440, y=u32 2 ("milliseconds to wait")) -> (x = y?=w438:bool)
        n281 = Select(t=T22."Disabled and Grayed Out" ("Disabled"), s=w438, f=T22."Enabled" ("Disabled")) -> (s? t:f=w435:T22)
        n282 = property on="Compression" class="Slide (strict)"("DisabledEnum"=w435) -> ()  [unwired: 2 in, 2 out]
      }
    }
  }
  n283 = while {
    tunnel: w38 -> [w443]
    i -> [w446]
    stop <- FALSE stop-if-true
    n284 = Wait (ms)(milliseconds to wait=u32 100) -> ()  [unwired: 1 out]
    n285 = case shown="\"Record\", Default" "Rec Mode" {
      tunnel: w446 -> [_ _ w461]
      tunnel: [u32 2829099 ("Base Color") u32 11141120 ("Target Color") w450] -> w442
      frame "Stop" {
        # "Reset the color, extra updates don't cost much"
      }
      frame "Record", Default {
      }
      frame "Playback" {
        # "Playback"
        n286 = Quotient & Remainder(x=w461, y=u32 50 ("milliseconds to wait")) -> (x-y*floor(x/y)=w457:u32)  [unwired: 1 out]
        n287 = Divide(x=w457, y=u32 50 ("milliseconds to wait")) -> (x/y=w454:dbl)
        n288 = Multiply(x=6.283185307179586, y=w454) -> (x*y=w459:dbl)
        n289 = Sine(x=w459) -> (sin(x)=w458:dbl)
        n290 = Absolute Value(x=w458) -> (abs(x)=w451:dbl)
        n291 = call "Interpolate RGB Color.vi"("Proportion"=w451, "Target Color"=u32 30976, "Base Color"=u32 2829099) -> ("Result Color"=w450:u32)  [unwired: 8 in]
      }
    }
    n292 = property class="Pane"(reference=w443, "PaneColor"=w442) -> ()  [unwired: 1 in, 2 out]
  }
  n293 = TCP Create Listener(10:u16 1741 ("timeout ms (25000)")) -> (3:w1:refnum<k5>)  [unwired: 4 in, 2 out]
  n294 = while {
    tunnel: w1 -> [w463]
    stop <- FALSE stop-if-true
    n295 = TCP Wait On Listener(11:w463) -> (4:w462:refnum<k5>)  [unwired: 3 in, 4 out]
    n296 = local write "TCP"(w462) -> ()
  }
  n297 = property on="On/Off" class="Bool (strict)"("Visible"=w6) -> ()  [unwired: 2 in, 2 out]
  n298 = property on="Motor" class="Clust (strict)"("Visible"=w6) -> ()  [unwired: 2 in, 2 out]
  n299 = property on="Progress" class="Clust (strict)"("Visible"=w6) -> ()  [unwired: 2 in, 2 out]
  n300 = property on="Test Ring" class="Ring (strict)"("Visible"=w6) -> ()  [unwired: 2 in, 2 out]
  n301 = property on="Rev/Fwd" class="Clust (strict)"("Visible"=w6) -> ()  [unwired: 2 in, 2 out]
  n302 = property on="Camera Settings" class="Clust (strict)"("Visible"=w6) -> ()  [unwired: 2 in, 2 out]
  n303 = local write "DB Camera Config"(w6) -> ()
  n304 = global write "WPI_DashboardLogging Global.vi" "Recording"(w32) -> ()
  n305 = local write "Rec Mode"(w32) -> ()
